vi "apply_noise_mask_to_image.vi"(10 "u8_ar_noise_mask in":u8[][](array[numeric]), 11 "Refnum in":T1) -> (1 "Image Pixels (U8)":u8[][](array[numeric]), 2 "Image Dst Out":T1, 3 "Refnum out":T1)   [LabVIEW 2011]
uses:
  <vilib>/vision/Image Controls.llb/IMAQ Image.ctl
  global_vars.vi
  <vilib>/vision/NI_Vision_Development_Module.lvlib
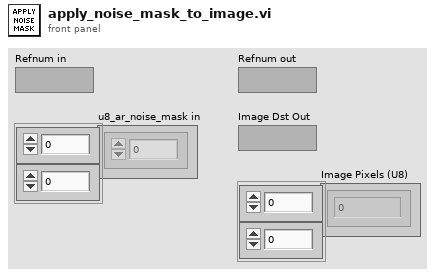
[diagram p1: front panel]
types:
  T1 = typedef "IMAQ Image.ctl" = refnum<image>
  T2 = typedef "Image Type" = u32
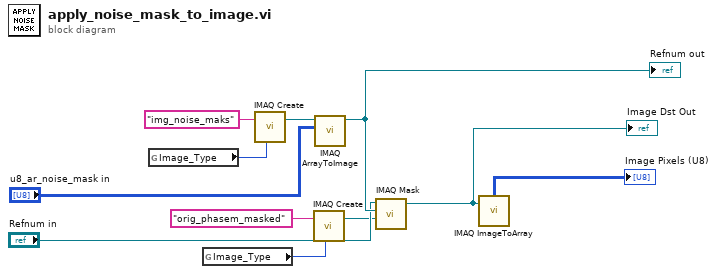
[diagram p0: block diagram]
diagram:
  n1 = global read "global_vars.vi" "Image_Type"() -> (w7:T2)
  n2 = global read "global_vars.vi" "Image_Type"() -> (w5:T2)
  n3 = call "IMAQ Create"("Image Name"="img_noise_maks", "Image Type"=w7) -> ("New Image"=w8:T1)  [unwired: 2 in, 2 out]
  n4 = call "IMAQ Create"("Image Name"="orig_phasem_masked", "Image Type"=w5) -> ("New Image"=w4:T1)  [unwired: 2 in, 2 out]
  n5 = call "IMAQ ArrayToImage"("Image Pixels (U8)"="u8_ar_noise_mask in", "Image"=w8) -> ("Image Out"=w11:T1)  [unwired: 8 in, 1 out]
  "Refnum out" <- w11
  n6 = call "IMAQ Mask"("Image Dst"=w4, "Image Mask"=w11, "Image Src"="Refnum in") -> ("Image Dst Out"=w2:T1)  [unwired: 2 in, 1 out]
  "Image Dst Out" <- w2
  n7 = call "IMAQ ImageToArray"("Image"=w2) -> ("Image Pixels (U8)"=→"Image Pixels (U8)":u8[][])  [unwired: 3 in, 4 out]
